vi "Autonomous Independent.vi"   [LabVIEW 2015]
doc: "This VI is called when autonomous begins, and will automatically be terminated when autonomous ends. You can carry out timed or sensor driven robot movement independently without needing to return to the caller."
uses:
  <vilib>/Rock Robotics/WPI/Solenoid/WPI_SolenoidValue.ctl
  <vilib>/Rock Robotics/WPI/Utilities/WPI_GetSetVariantRefNum.vi
  Robot Global Data.vi
  <vilib>/Rock Robotics/WPI/Solenoid/WPI_SolenoidSetEnum.vi
panel:
  # "Be sure to right-click and choose Data Operations>>Make Current Value default if you want to save the array values with the VI"
types:
  T1 = typedef "WPI_JoystickDevRef.ctl" = cluster{"Device":T2}
  T2 = typedef "WPI_JoystickDeviceEnum.ctl" = enum16{"USB 0", "USB 1", "USB 2", "USB 3", "USB 4", "USB 5"}
  T3 = typedef "WPI_SwitchDevRef.ctl" = cluster{"DevStatus":errorcluster, "DIO Channel":T4, "CntIndex":T5, "Normally Closed":bool}
  T4 = typedef "FPGA_DIOChannel.ctl" = enum8{"DIO 0", "DIO 1", "DIO 2", "DIO 3", "DIO 4", "DIO 5", "DIO 6", "DIO 7", "DIO 8", "DIO 9", "DIO MXP 0", "DIO MXP 1", "DIO MXP 2", "DIO MXP 3", "DIO MXP 4", "DIO MXP 5", "DIO MXP 6", "DIO MXP 7", "DIO MXP 8", "DIO MXP 9", "DIO MXP 10", "DIO MXP 11", "DIO MXP 12", "DIO MXP 13", "DIO MXP 14", "DIO MXP 15", "Invalid"}
  T5 = typedef "FPGA_CounterCtrSystemIndex.ctl" = enum8{"Ctr 0", "Ctr 1", "Ctr 2", "Ctr 3", "Ctr 4", "Ctr 5", "Ctr 6", "Ctr 7", "Invalid"}
  T6 = typedef "WPI_SolenoidValue.ctl" = enum16{"Off", "On", "Forward", "Reverse"}
  T7 = enum16{"No pot 1 bin", "3 Tote Spinny", "2 Tote Middle", "1 Bin", "1 Tote", "Drive", "3 Tote"}
  T8 = typedef "WPI_SolenoidDevRef.ctl" = cluster{"DevStatus":errorcluster, "Pneumatics Control Module":u8, "Forward Solenoid Channel":T9, "Reverse Solenoid Channel":T9}
  T9 = typedef "WPI_SolenoidChannel.ctl" = enum8{"Solenoid 0", "Solenoid 1", "Solenoid 2", "Solenoid 3", "Solenoid 4", "Solenoid 5", "Solenoid 6", "Solenoid 7", "Invalid"}
  T10 = typedef "WPI_MotorControlDeviceRef.ctl" = cluster{"DeviceStatus":errorcluster, "Type":T11, "PWM":cluster{"PWM Channel":T12, "DeadBand":T13}, "CAN":cluster{"Device Number":u8, "Control Mode":T14, "Semaphore":T15, "Max Vout":dbl, "TalonSRX Control Mode":T16}, "Invert":bool}
  T11 = typedef "WPI_MotorControlType.ctl" = enum16{"PWM", "CAN", "CANTalonSRX"}
  T12 = typedef "FPGA_DIOPWMChannel.ctl" = enum8{"PWM 0", "PWM 1", "PWM 2", "PWM 3", "PWM 4", "PWM 5", "PWM 6", "PWM 7", "PWM 8", "PWM 9", "PWM MXP 0", "PWM MXP 1", "PWM MXP 2", "PWM MXP 3", "PWM MXP 4", "PWM MXP 5", "PWM MXP 6", "PWM MXP 7", "PWM MXP 8", "PWM MXP 9", "Invalid"}
  T13 = typedef "WPI_PWMDeadband.ctl" = cluster{"Name":string, "maxPositivePwm":i32, "minPositivePwm":i32, "centerPwm":i32, "maxNegativePwm":i32, "minNegativePwm":i32, "angularRange":u16}
  T14 = typedef "WPI_CANJaguar_ControlMode.ctl" = enum8{"Percent VBus", "Current", "Speed", "Position", "Voltage"}
  T15 = typedef "Semaphore RefNum" = refnum<k1>
  T16 = typedef "WPI_CANTalonSRX_APIControlMode.ctl" = enum8{"Percent VBus", "Speed", "Position", "Slave", "Unchanged / Invalid", "Voltage Compensation", "Current", "Motion Profile"}
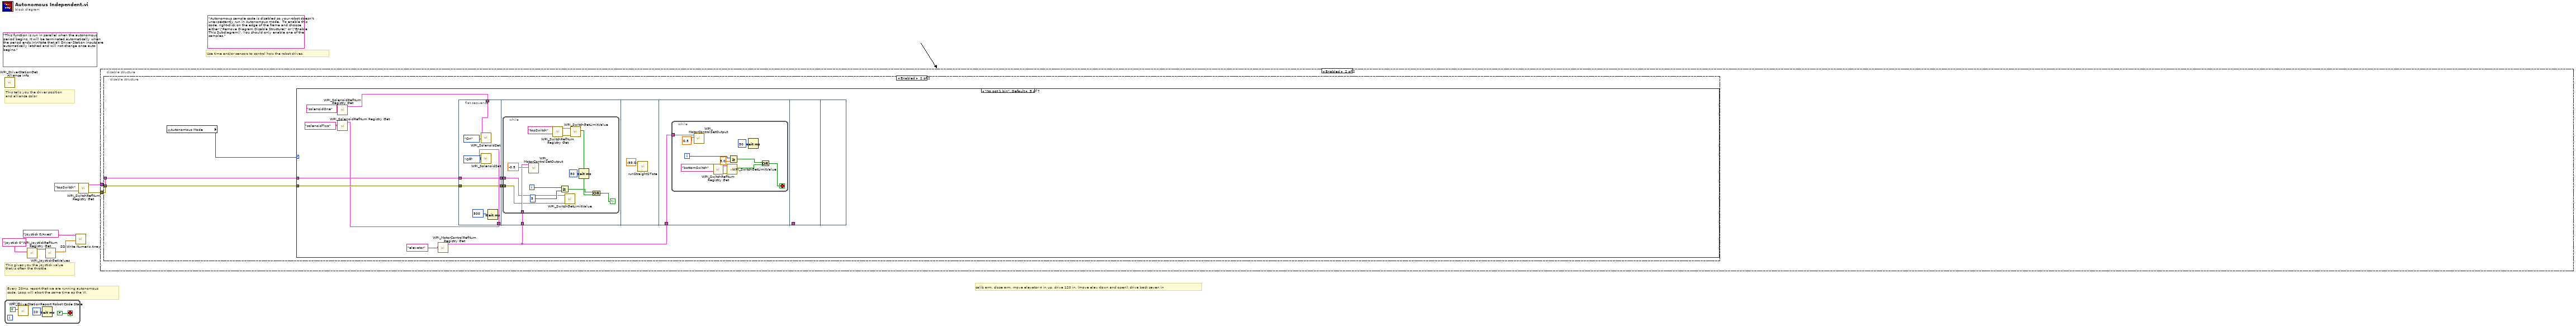
[diagram p0: block diagram]
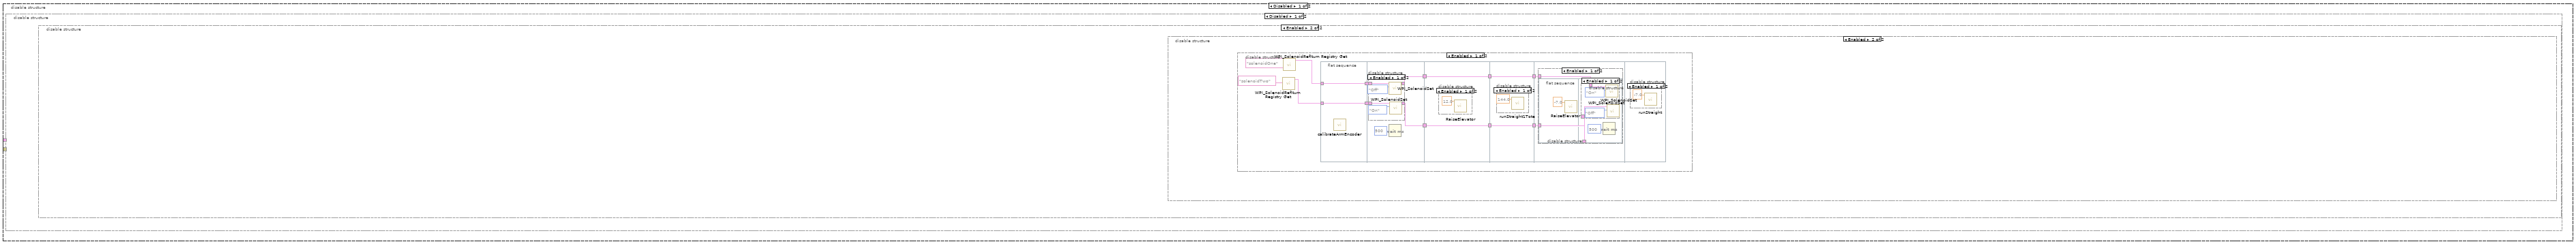
[diagram p2: hidden frame]
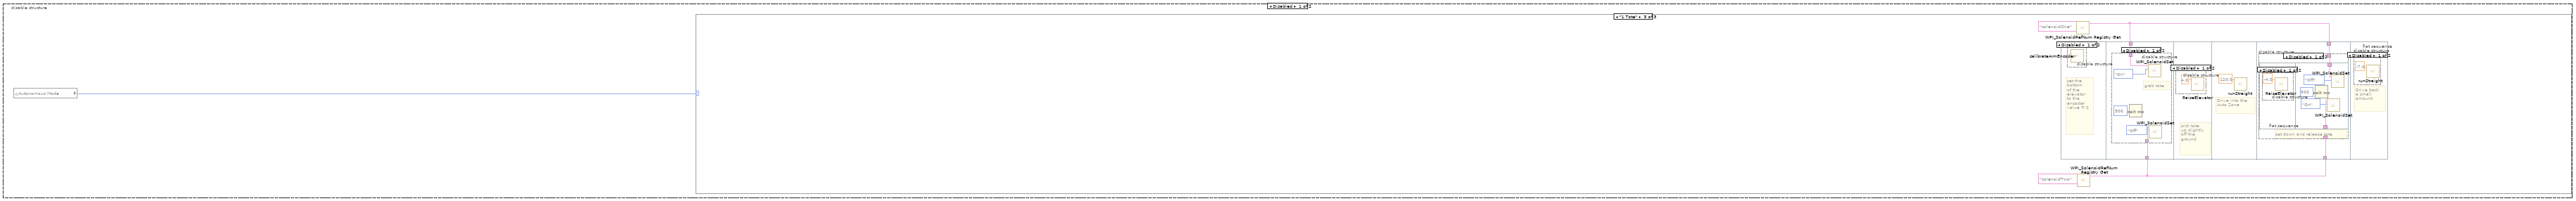
[diagram p3: hidden frame]
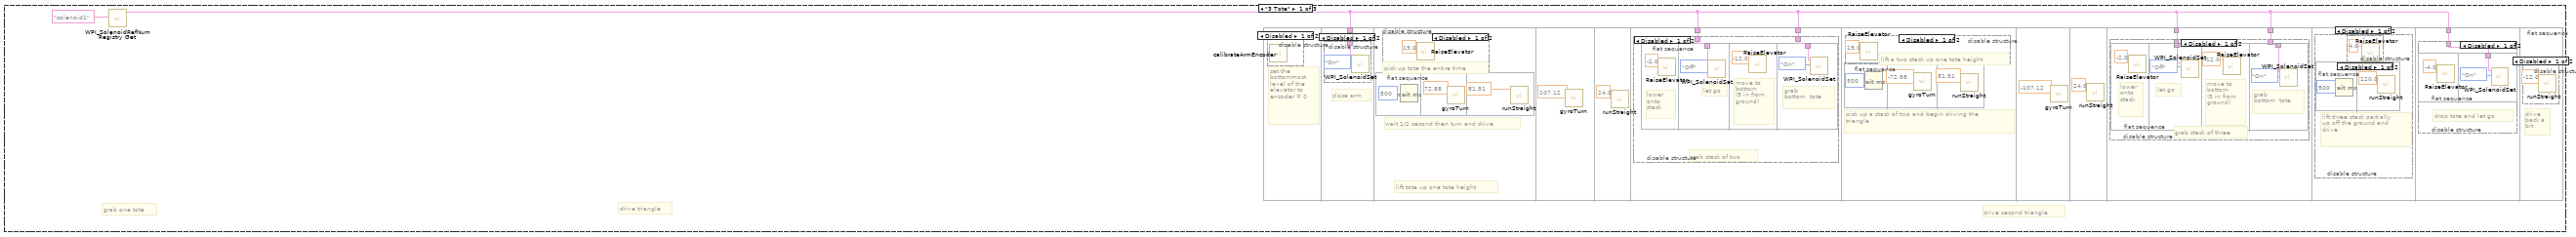
[diagram p4: hidden frame]
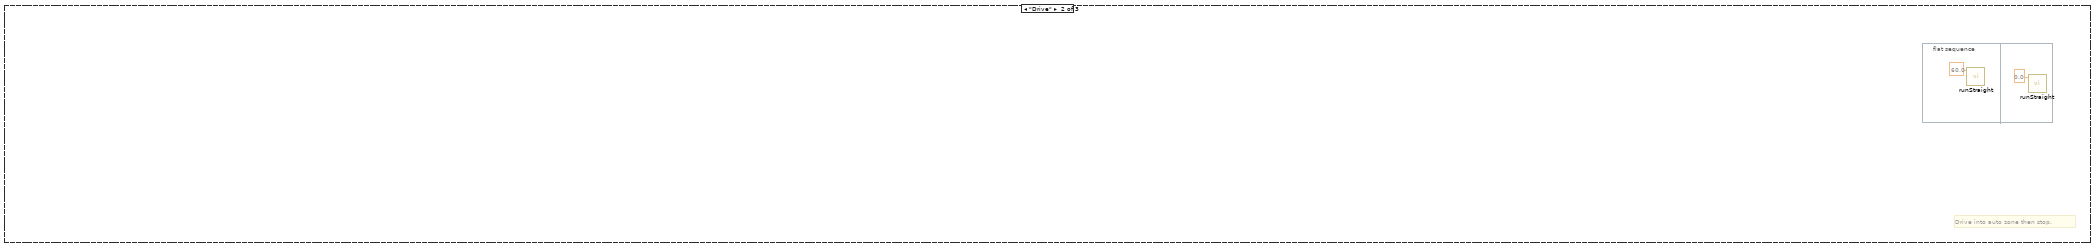
[diagram p15: hidden frame]
diagram:
  (unwired) "Autonomous sample code is disabled so your robot doesn't unexpectantly run in Autonomous mode.  To enable this code, right-click on the edge of the frame and choose either \"Remove Diagram Disable Structure\" or \"Enable This Subdiagram\". You should only enable one of the samples."
  (unwired) "This function is run in parallel when the autonomous period begins. It will be terminated automatically when the period ends.\n\nNote that all Driver Station inputs are automatically latched and will not change once auto begins."
  # "calib arm, close arm, move elevator 4 in up, drive 120 in, (move elev down and open), drive back seven in"
  # "Every 20ms, report that we are running autonomous\ncode. Loop will abort the same time as the VI."
  # "This gives you the joystick value\nthat is often the throttle"
  # "Use time and/or sensors to control how the robot drives."
  # "This tells you the driver position\nand alliance color"
  n1 = while {
    stop <- FALSE stop-if-true
    n2 = call <vilib>:"WPI_DriverStationReport Robot Code State.vi"("Autonomous"=TRUE) -> ()  [unwired: 10 in, 1 out]
    n3 = Wait (ms)(milliseconds to wait=u32 20) -> ()  [unwired: 1 out]
  }
  n4 = call <vilib>:"WPI_DriverStationGet Alliance Info.vi"() -> ()  [unwired: 12 out]
  n5 = call <vilib>:"WPI_JoystickRefNum Registry Get.vi"("refnum name"="Joystick 0") -> ("JoystickDevRef"=w6:T1)  [unwired: 1 in, 9 out]
  n6 = call <vilib>:"WPI_JoystickGetValues.vi"("JoystickDevRef"=w6) -> ("Axes"=w4:dbl[])  [unwired: 6 in, 4 out]
  n7 = call <vilib>:"SD Write Numeric Array.vi"("Numeric Array"=w4, "Name"="Joystick 0/Axes") -> ()  [unwired: 8 in, 2 out]
  n8 = call <vilib>:"WPI_SwitchRefNum Registry Get.vi"("refnum name"="topSwitch") -> ("error out"=w1:errorcluster, "SwitchDevRef"=w2:T3)  [unwired: 9 in]
  n9 = disable-structure shown="Enabled" {
    disable-tunnel: w2 -> [_ w201]
    disable-tunnel: w1 -> [_ w200]
    frame Disabled {
      n10 = disable-structure shown="Disabled" {
        frame Disabled {
          n11 = disable-structure shown="Enabled" {
            frame Disabled {
              n12 = global read "Robot Global Data.vi" "Autonomous Mode"() -> (w11:T7)
              n13 = case shown="\"1 Tote\"" w11 {
                frame "3 Tote" {
                  # "drive triangle"
                  # "drive second triangle"
                  # "grab one tote"
                  n14 = call <vilib>:"WPI_SolenoidRefNum Registry Get.vi"("refnum name"="solenoid1") -> ("SolenoidDevRef"=w13:T8)  [unwired: 9 in, 1 out]
                  n15 = flat-sequence {
                    tunnel: w13 -> [w14]
                    tunnel: w13 -> [w24]
                    tunnel: w13 -> [w23]
                    tunnel: w13 -> [w40]
                    tunnel: w13 -> [w39]
                    tunnel: w13 -> [w52]
                    frame #0 {
                      # "set the \nbottommost\nlevel of the \nelevator to \nencoder = 0"
                      n16 = disable-structure shown="Disabled" {
                        frame Disabled {
                          n17 = call "calibrateArmEncoder.vi"() -> ()  [unwired: 12 in]
                        }
                        frame Enabled {
                        }
                      }
                    }
                    frame #1 {
                      # "close arm"
                      n18 = disable-structure shown="Disabled" {
                        disable-tunnel: w14 -> [w15 _]
                        frame Disabled {
                          n19 = call-poly <vilib>:"WPI_SolenoidSet.vi"("Value"=WPI_SolenoidValue."On", "SolenoidDevRef"=w15) -> ()  [unwired: 8 in, 2 out]
                        }
                        frame Enabled {
                        }
                      }
                    }
                    frame #2 {
                      # "lift tote up one tote height"
                      # "wait 1/2 second then turn and drive"
                      n20 = flat-sequence {
                        frame #0 {
                          n21 = Wait (ms)(milliseconds to wait=u32 500) -> ()  [unwired: 1 out]
                        }
                        frame #1 {
                          n22 = call "gyroTurn.vi"("Angle"=72.88) -> ()  [unwired: 11 in]
                        }
                        frame #2 {
                          n23 = call "runStraight.vi"("Distance In"=81.51) -> ()  [unwired: 11 in]
                        }
                      }
                      n24 = disable-structure shown="Disabled" {
                        frame Disabled {
                          # "pick up tote the entire time"
                          n25 = call "RaiseElevator.vi"("Distance"=19.0) -> ()  [unwired: 11 in]
                        }
                        frame Enabled {
                        }
                      }
                    }
                    frame #3 {
                      n26 = call "gyroTurn.vi"("Angle"=107.12) -> ()  [unwired: 11 in]
                    }
                    frame #4 {
                      n27 = call "runStraight.vi"("Distance In"=24.0) -> ()  [unwired: 11 in]
                    }
                    frame #5 {
                      n28 = disable-structure shown="Disabled" {
                        disable-tunnel: w24 -> [w26 _]
                        disable-tunnel: w23 -> [w25 _]
                        frame Disabled {
                          # "grab stack of two"
                          n29 = flat-sequence {
                            tunnel: w26 -> [w28]
                            tunnel: w25 -> [w31]
                            frame #0 {
                              # "lower onto\nstack"
                              n30 = call "RaiseElevator.vi"("Distance"=-2.0) -> ()  [unwired: 11 in]
                            }
                            frame #1 {
                              # "let go"
                              n31 = call-poly <vilib>:"WPI_SolenoidSet.vi"("Value"=WPI_SolenoidValue."Off", "SolenoidDevRef"=w28) -> ()  [unwired: 8 in, 2 out]
                            }
                            frame #2 {
                              # "move to\nbottom \n(5 in from\nground)"
                              n32 = call "RaiseElevator.vi"("Distance"=-12.0) -> ()  [unwired: 11 in]
                            }
                            frame #3 {
                              # "grab \nbottom  tote"
                              n33 = call-poly <vilib>:"WPI_SolenoidSet.vi"("Value"=WPI_SolenoidValue."On", "SolenoidDevRef"=w31) -> ()  [unwired: 8 in, 2 out]
                            }
                          }
                        }
                        frame Enabled {
                        }
                      }
                    }
                    frame #6 {
                      # "pick up a stack of two and begin driving the \ntriangle"
                      n34 = flat-sequence {
                        frame #0 {
                          n35 = Wait (ms)(milliseconds to wait=u32 500) -> ()  [unwired: 1 out]
                        }
                        frame #1 {
                          n36 = call "gyroTurn.vi"("Angle"=-72.88) -> ()  [unwired: 11 in]
                        }
                        frame #2 {
                          n37 = call "runStraight.vi"("Distance In"=81.51) -> ()  [unwired: 11 in]
                        }
                      }
                      n38 = disable-structure shown="Disabled" {
                        frame Disabled {
                          # "lift a two stack up one tote height"
                          n39 = call "RaiseElevator.vi"("Distance"=19.0) -> ()  [unwired: 11 in]
                        }
                        frame Enabled {
                        }
                      }
                    }
                    frame #7 {
                      n40 = call "gyroTurn.vi"("Angle"=-107.12) -> ()  [unwired: 11 in]
                    }
                    frame #8 {
                      n41 = call "runStraight.vi"("Distance In"=24.0) -> ()  [unwired: 11 in]
                    }
                    frame #9 {
                      n42 = disable-structure shown="Disabled" {
                        disable-tunnel: w40 -> [w42 _]
                        disable-tunnel: w39 -> [w41 _]
                        frame Disabled {
                          # "grab stack of three"
                          n43 = flat-sequence {
                            tunnel: w42 -> [w44]
                            tunnel: w41 -> [w47]
                            frame #0 {
                              # "lower\nonto\nstack"
                              n44 = call "RaiseElevator.vi"("Distance"=-2.0) -> ()  [unwired: 11 in]
                            }
                            frame #1 {
                              # "let go"
                              n45 = call-poly <vilib>:"WPI_SolenoidSet.vi"("Value"=WPI_SolenoidValue."Off", "SolenoidDevRef"=w44) -> ()  [unwired: 8 in, 2 out]
                            }
                            frame #2 {
                              # "move to\nbottom \n(5 in from\nground)"
                              n46 = call "RaiseElevator.vi"("Distance"=-12.0) -> ()  [unwired: 11 in]
                            }
                            frame #3 {
                              # "grab \nbottom  tote"
                              n47 = call-poly <vilib>:"WPI_SolenoidSet.vi"("Value"=WPI_SolenoidValue."On", "SolenoidDevRef"=w47) -> ()  [unwired: 8 in, 2 out]
                            }
                          }
                        }
                        frame Enabled {
                        }
                      }
                    }
                    frame #10 {
                      n48 = disable-structure shown="Disabled" {
                        frame Disabled {
                          # "lift three stack partially \nup off the ground and \ndrive"
                          n49 = flat-sequence {
                            frame #0 {
                              n50 = Wait (ms)(milliseconds to wait=u32 500) -> ()  [unwired: 1 out]
                            }
                            frame #1 {
                              n51 = call "runStraight.vi"("Distance In"=120.0) -> ()  [unwired: 11 in]
                            }
                          }
                          n52 = disable-structure shown="Disabled" {
                            frame Disabled {
                              n53 = call "RaiseElevator.vi"("Distance"=4.0) -> ()  [unwired: 11 in]
                            }
                            frame Enabled {
                            }
                          }
                        }
                        frame Enabled {
                        }
                      }
                    }
                    frame #11 {
                      n54 = disable-structure shown="Disabled" {
                        disable-tunnel: w52 -> [w53 _]
                        frame Disabled {
                          # "drop tote and let go"
                          n55 = flat-sequence {
                            tunnel: w53 -> [w55]
                            frame #0 {
                              n56 = call "RaiseElevator.vi"("Distance"=-4.0) -> ()  [unwired: 11 in]
                            }
                            frame #1 {
                              n57 = call-poly <vilib>:"WPI_SolenoidSet.vi"("Value"=WPI_SolenoidValue."On", "SolenoidDevRef"=w55) -> ()  [unwired: 8 in, 2 out]
                            }
                          }
                        }
                        frame Enabled {
                        }
                      }
                    }
                    frame #12 {
                      # "drive \nback a \nbit"
                      n58 = disable-structure shown="Disabled" {
                        frame Disabled {
                          n59 = call "runStraight.vi"("Distance In"=-12.0) -> ()  [unwired: 11 in]
                        }
                        frame Enabled {
                        }
                      }
                    }
                  }
                }
                frame "Drive" {
                  # "Drive into auto zone then stop."
                  n60 = flat-sequence {
                    frame #0 {
                      n61 = call "runStraight.vi"("Distance In"=60.0) -> ()  [unwired: 11 in]
                    }
                    frame #1 {
                      n62 = call "runStraight.vi"("Distance In"=0.0) -> ()  [unwired: 11 in]
                    }
                  }
                }
                frame "1 Tote" {
                  n63 = flat-sequence {
                    tunnel: w62 -> [w65]
                    tunnel: w60 -> [w64]
                    tunnel: w62 -> [w74]
                    tunnel: w60 -> [w73]
                    frame #0 {
                      # "set the \nbottom\nof the\nelevator\nto the\nencoder\nvalue = 0"
                      n64 = disable-structure shown="Disabled" {
                        frame Disabled {
                          n65 = call "calibrateArmEncoder.vi"() -> ()  [unwired: 12 in]
                        }
                        frame Enabled {
                        }
                      }
                    }
                    frame #1 {
                      n66 = disable-structure shown="Disabled" {
                        disable-tunnel: w65 -> [w70 _]
                        disable-tunnel: w64 -> [w67 _]
                        frame Disabled {
                          # "grab tote"
                          n67 = Wait (ms)(milliseconds to wait=u32 500) -> ()  [unwired: 1 out]
                          n68 = call-poly <vilib>:"WPI_SolenoidSet.vi"("Value"=WPI_SolenoidValue."On", "SolenoidDevRef"=w70) -> ()  [unwired: 8 in, 2 out]
                          n69 = call-poly <vilib>:"WPI_SolenoidSet.vi"("Value"=WPI_SolenoidValue."Off", "SolenoidDevRef"=w67) -> ()  [unwired: 8 in, 2 out]
                        }
                        frame Enabled {
                        }
                      }
                    }
                    frame #2 {
                      # "pick tote\nup slightly\noff the \nground"
                      n70 = disable-structure shown="Disabled" {
                        frame Disabled {
                          n71 = call "RaiseElevator.vi"("Distance"=4.0) -> ()  [unwired: 11 in]
                        }
                        frame Enabled {
                        }
                      }
                    }
                    frame #3 {
                      # "Drive into the\nAuto Zone"
                      n72 = call "runStraight.vi"("Distance In"=120.0) -> ()  [unwired: 11 in]
                    }
                    frame #4 {
                      n73 = disable-structure shown="Disabled" {
                        disable-tunnel: w74 -> [w76 _]
                        disable-tunnel: w73 -> [w75 _]
                        frame Disabled {
                          # "set down and release tote"
                          n74 = flat-sequence {
                            tunnel: w76 -> [w81]
                            tunnel: w75 -> [w79]
                            frame #0 {
                              n75 = disable-structure shown="Disabled" {
                                frame Disabled {
                                n76 = call "RaiseElevator.vi"("Distance"=-4.0) -> ()  [unwired: 11 in]
                                }
                                frame Enabled {
                                }
                              }
                            }
                            frame #1 {
                              n77 = Wait (ms)(milliseconds to wait=u32 500) -> ()  [unwired: 1 out]
                              n78 = call-poly <vilib>:"WPI_SolenoidSet.vi"("Value"=WPI_SolenoidValue."On", "SolenoidDevRef"=w79) -> ()  [unwired: 8 in, 2 out]
                              n79 = call-poly <vilib>:"WPI_SolenoidSet.vi"("Value"=WPI_SolenoidValue."Off", "SolenoidDevRef"=w81) -> ()  [unwired: 8 in, 2 out]
                            }
                          }
                        }
                        frame Enabled {
                        }
                      }
                    }
                    frame #5 {
                      # "Drive back\na small \namount"
                      n80 = disable-structure shown="Disabled" {
                        frame Disabled {
                          n81 = call "runStraight.vi"("Distance In"=-7.0) -> ()  [unwired: 11 in]
                        }
                        frame Enabled {
                        }
                      }
                    }
                  }
                  n82 = call <vilib>:"WPI_SolenoidRefNum Registry Get.vi"("refnum name"="solenoidOne") -> ("SolenoidDevRef"=w62:T8)  [unwired: 9 in, 1 out]
                  n83 = call <vilib>:"WPI_SolenoidRefNum Registry Get.vi"("refnum name"="solenoidTwo") -> ("SolenoidDevRef"=w60:T8)  [unwired: 9 in, 1 out]
                }
              }
            }
            frame Enabled {
              n84 = disable-structure shown="Enabled" {
                frame Disabled {
                  # "drive triangle"
                  # "drive second triangle"
                  # "grab one tote"
                  n85 = call <vilib>:"WPI_SolenoidRefNum Registry Get.vi"("refnum name"="solenoid1") -> ("SolenoidDevRef"=w85:T8)  [unwired: 9 in, 1 out]
                  n86 = flat-sequence {
                    tunnel: w85 -> [w86]
                    tunnel: w85 -> [w96]
                    tunnel: w85 -> [w95]
                    tunnel: w85 -> [w112]
                    tunnel: w85 -> [w111]
                    tunnel: w85 -> [w124]
                    frame #0 {
                      # "set the \nbottommost\nlevel of the \nelevator to \nencoder = 0"
                      n87 = disable-structure shown="Disabled" {
                        frame Disabled {
                          n88 = call "calibrateArmEncoder.vi"() -> ()  [unwired: 12 in]
                        }
                        frame Enabled {
                        }
                      }
                    }
                    frame #1 {
                      # "close arm"
                      n89 = disable-structure shown="Disabled" {
                        disable-tunnel: w86 -> [w87 _]
                        frame Disabled {
                          n90 = call-poly <vilib>:"WPI_SolenoidSet.vi"("Value"=WPI_SolenoidValue."On", "SolenoidDevRef"=w87) -> ()  [unwired: 8 in, 2 out]
                        }
                        frame Enabled {
                        }
                      }
                    }
                    frame #2 {
                      # "lift tote up one tote height"
                      # "wait 1/2 second then turn and drive"
                      n91 = flat-sequence {
                        frame #0 {
                          n92 = Wait (ms)(milliseconds to wait=u32 500) -> ()  [unwired: 1 out]
                        }
                        frame #1 {
                          n93 = call "gyroTurn.vi"("Angle"=-72.88) -> ()  [unwired: 11 in]
                        }
                        frame #2 {
                          n94 = call "runStraight.vi"("Distance In"=81.51) -> ()  [unwired: 11 in]
                        }
                      }
                      n95 = disable-structure shown="Disabled" {
                        frame Disabled {
                          # "pick up tote the entire time"
                          n96 = call "RaiseElevator.vi"("Distance"=19.0) -> ()  [unwired: 11 in]
                        }
                        frame Enabled {
                        }
                      }
                    }
                    frame #3 {
                      n97 = call "gyroTurn.vi"("Angle"=-107.12) -> ()  [unwired: 11 in]
                    }
                    frame #4 {
                      n98 = call "runStraight.vi"("Distance In"=24.0) -> ()  [unwired: 11 in]
                    }
                    frame #5 {
                      n99 = disable-structure shown="Disabled" {
                        disable-tunnel: w96 -> [w98 _]
                        disable-tunnel: w95 -> [w97 _]
                        frame Disabled {
                          # "grab stack of two"
                          n100 = flat-sequence {
                            tunnel: w98 -> [w100]
                            tunnel: w97 -> [w103]
                            frame #0 {
                              # "lower onto\nstack"
                              n101 = call "RaiseElevator.vi"("Distance"=-2.0) -> ()  [unwired: 11 in]
                            }
                            frame #1 {
                              # "let go"
                              n102 = call-poly <vilib>:"WPI_SolenoidSet.vi"("Value"=WPI_SolenoidValue."Off", "SolenoidDevRef"=w100) -> ()  [unwired: 8 in, 2 out]
                            }
                            frame #2 {
                              # "move to\nbottom \n(5 in from\nground)"
                              n103 = call "RaiseElevator.vi"("Distance"=-12.0) -> ()  [unwired: 11 in]
                            }
                            frame #3 {
                              # "grab \nbottom  tote"
                              n104 = call-poly <vilib>:"WPI_SolenoidSet.vi"("Value"=WPI_SolenoidValue."On", "SolenoidDevRef"=w103) -> ()  [unwired: 8 in, 2 out]
                            }
                          }
                        }
                        frame Enabled {
                        }
                      }
                    }
                    frame #6 {
                      # "pick up a stack of two and begin driving the \ntriangle"
                      n105 = flat-sequence {
                        frame #0 {
                          n106 = Wait (ms)(milliseconds to wait=u32 500) -> ()  [unwired: 1 out]
                        }
                        frame #1 {
                          n107 = call "gyroTurn.vi"("Angle"=72.88) -> ()  [unwired: 11 in]
                        }
                        frame #2 {
                          n108 = call "runStraight.vi"("Distance In"=81.51) -> ()  [unwired: 11 in]
                        }
                      }
                      n109 = disable-structure shown="Disabled" {
                        frame Disabled {
                          # "lift a two stack up one tote height"
                          n110 = call "RaiseElevator.vi"("Distance"=19.0) -> ()  [unwired: 11 in]
                        }
                        frame Enabled {
                        }
                      }
                    }
                    frame #7 {
                      n111 = call "gyroTurn.vi"("Angle"=107.12) -> ()  [unwired: 11 in]
                    }
                    frame #8 {
                      n112 = call "runStraight.vi"("Distance In"=24.0) -> ()  [unwired: 11 in]
                    }
                    frame #9 {
                      n113 = disable-structure shown="Disabled" {
                        disable-tunnel: w112 -> [w114 _]
                        disable-tunnel: w111 -> [w113 _]
                        frame Disabled {
                          # "grab stack of three"
                          n114 = flat-sequence {
                            tunnel: w114 -> [w116]
                            tunnel: w113 -> [w119]
                            frame #0 {
                              # "lower\nonto\nstack"
                              n115 = call "RaiseElevator.vi"("Distance"=-2.0) -> ()  [unwired: 11 in]
                            }
                            frame #1 {
                              # "let go"
                              n116 = call-poly <vilib>:"WPI_SolenoidSet.vi"("Value"=WPI_SolenoidValue."Off", "SolenoidDevRef"=w116) -> ()  [unwired: 8 in, 2 out]
                            }
                            frame #2 {
                              # "move to\nbottom \n(5 in from\nground)"
                              n117 = call "RaiseElevator.vi"("Distance"=-12.0) -> ()  [unwired: 11 in]
                            }
                            frame #3 {
                              # "grab \nbottom  tote"
                              n118 = call-poly <vilib>:"WPI_SolenoidSet.vi"("Value"=WPI_SolenoidValue."On", "SolenoidDevRef"=w119) -> ()  [unwired: 8 in, 2 out]
                            }
                          }
                        }
                        frame Enabled {
                        }
                      }
                    }
                    frame #10 {
                      n119 = disable-structure shown="Disabled" {
                        frame Disabled {
                          # "lift three stack partially \nup off the ground and \ndrive"
                          n120 = flat-sequence {
                            frame #0 {
                              n121 = Wait (ms)(milliseconds to wait=u32 500) -> ()  [unwired: 1 out]
                            }
                            frame #1 {
                              n122 = call "runStraight.vi"("Distance In"=120.0) -> ()  [unwired: 11 in]
                            }
                          }
                          n123 = disable-structure shown="Disabled" {
                            frame Disabled {
                              n124 = call "RaiseElevator.vi"("Distance"=4.0) -> ()  [unwired: 11 in]
                            }
                            frame Enabled {
                            }
                          }
                        }
                        frame Enabled {
                        }
                      }
                    }
                    frame #11 {
                      n125 = disable-structure shown="Disabled" {
                        disable-tunnel: w124 -> [w125 _]
                        frame Disabled {
                          # "drop tote and let go"
                          n126 = flat-sequence {
                            tunnel: w125 -> [w127]
                            frame #0 {
                              n127 = call "RaiseElevator.vi"("Distance"=-4.0) -> ()  [unwired: 11 in]
                            }
                            frame #1 {
                              n128 = call-poly <vilib>:"WPI_SolenoidSet.vi"("Value"=WPI_SolenoidValue."On", "SolenoidDevRef"=w127) -> ()  [unwired: 8 in, 2 out]
                            }
                          }
                        }
                        frame Enabled {
                        }
                      }
                    }
                    frame #12 {
                      # "drive \nback a \nbit"
                      n129 = disable-structure shown="Disabled" {
                        frame Disabled {
                          n130 = call "runStraight.vi"("Distance In"=-12.0) -> ()  [unwired: 11 in]
                        }
                        frame Enabled {
                        }
                      }
                    }
                  }
                }
                frame Enabled {
                  n131 = disable-structure shown="Enabled" {
                    frame Enabled {
                      n132 = call <vilib>:"WPI_SolenoidRefNum Registry Get.vi"("refnum name"="solenoidTwo") -> ("SolenoidDevRef"=w132:T8)  [unwired: 9 in, 1 out]
                      n133 = call <vilib>:"WPI_SolenoidRefNum Registry Get.vi"("refnum name"="solenoidOne") -> ("SolenoidDevRef"=w133:T8)  [unwired: 9 in, 1 out]
                      n134 = flat-sequence {
                        tunnel: w132 -> [w142]
                        tunnel: w133 -> [w143]
                        tunnel: [w143] -> w141
                        tunnel: [w142] -> w140
                        tunnel: [w146] -> w139
                        tunnel: [w145] -> w138
                        tunnel: w141 -> [w148]
                        tunnel: w140 -> [w147]
                        tunnel: [w156] -> w137
                        tunnel: w139 -> [w156]
                        tunnel: [w155] -> w136
                        tunnel: w138 -> [w155]
                        tunnel: [w159] -> w135
                        tunnel: w137 -> [w159]
                        tunnel: [w158] -> w134
                        tunnel: w136 -> [w158]
                        tunnel: w135 -> [w162]
                        tunnel: w134 -> [w161]
                        frame #0 {
                          n135 = call "calibrateArmEncoder.vi"() -> ()  [unwired: 12 in]
                        }
                        frame #1 {
                          n136 = disable-structure shown="Enabled" {
                            disable-tunnel: w148 -> [w154 _]
                            disable-tunnel: w147 -> [w153 _]
                            disable-tunnel: [w150 _] -> w146
                            disable-tunnel: [w149 _] -> w145
                            frame Enabled {
                              n137 = call-poly <vilib>:"WPI_SolenoidSet.vi"("Value"=WPI_SolenoidValue."Off", "SolenoidDevRef"=w154) -> ("SolenoidDevRef"=w150:T8)  [unwired: 8 in, 1 out]
                              n138 = call-poly <vilib>:"WPI_SolenoidSet.vi"("Value"=WPI_SolenoidValue."On", "SolenoidDevRef"=w153) -> ("SolenoidDevRef"=w149:T8)  [unwired: 8 in, 1 out]
                            }
                            frame Disabled {
                            }
                          }
                          n139 = Wait (ms)(milliseconds to wait=u32 500) -> ()  [unwired: 1 out]
                        }
                        frame #2 {
                          n140 = disable-structure shown="Enabled" {
                            frame Enabled {
                              n141 = call "RaiseElevator.vi"("Distance"=12.0) -> ()  [unwired: 11 in]
                            }
                            frame Disabled {
                            }
                          }
                        }
                        frame #3 {
                          n142 = disable-structure shown="Enabled" {
                            frame Enabled {
                              n143 = call "runStraight1Tote.vi"("Distance In"=144.0) -> ()  [unwired: 11 in]
                            }
                            frame Disabled {
                            }
                          }
                        }
                        frame #4 {
                          n144 = disable-structure shown="Enabled" {
                            disable-tunnel: w162 -> [w164 _]
                            disable-tunnel: w161 -> [w163 _]
                            frame Enabled {
                              n145 = flat-sequence {
                                tunnel: w164 -> [w168]
                                tunnel: w163 -> [w167]
                                frame #0 {
                                n146 = call "RaiseElevator.vi"("Distance"=-7.0) -> ()  [unwired: 11 in]
                                }
                                frame #1 {
                                n147 = disable-structure shown="Enabled" {
                                disable-tunnel: w168 -> [w170 _]
                                disable-tunnel: w167 -> [w169 _]
                                frame Enabled {
                                n148 = call-poly <vilib>:"WPI_SolenoidSet.vi"("Value"=WPI_SolenoidValue."On", "SolenoidDevRef"=w170) -> ()  [unwired: 8 in, 2 out]
                                n149 = call-poly <vilib>:"WPI_SolenoidSet.vi"("Value"=WPI_SolenoidValue."Off", "SolenoidDevRef"=w169) -> ()  [unwired: 8 in, 2 out]
                                }
                                frame Disabled {
                                }
                                }
                                n150 = Wait (ms)(milliseconds to wait=u32 500) -> ()  [unwired: 1 out]
                                }
                              }
                            }
                            frame Disabled {
                            }
                          }
                        }
                        frame #5 {
                          n151 = disable-structure shown="Enabled" {
                            frame Enabled {
                              n152 = call "runStraight.vi"("Distance In"=-7.0) -> ()  [unwired: 11 in]
                            }
                            frame Disabled {
                            }
                          }
                        }
                      }
                    }
                    frame Disabled {
                      n153 = flat-sequence {
                        frame #0 {
                          n154 = call "gyroTurn.vi"("Angle"=90.0) -> ()  [unwired: 11 in]
                        }
                      }
                    }
                  }
                }
              }
            }
          }
        }
        frame Enabled {
          n155 = call <vilib>:"WPI_SolenoidRefNum Registry Get.vi"("refnum name"="solenoidTwo") -> ("SolenoidDevRef"=w176:T8)  [unwired: 9 in, 1 out]
          n156 = call <vilib>:"WPI_SolenoidRefNum Registry Get.vi"("refnum name"="solenoidOne") -> ("SolenoidDevRef"=w175:T8)  [unwired: 9 in, 1 out]
          n157 = flat-sequence {
            tunnel: w176 -> [w185]
            tunnel: w175 -> [w184]
            tunnel: w175 -> [w192]
            tunnel: w176 -> [w191]
            frame #0 {
              n158 = call "calibrateArmEncoder.vi"() -> ()  [unwired: 12 in]
            }
            frame #1 {
              # "raise elevator"
              n159 = call "RaiseElevator.vi"("Distance"=14.0) -> ()  [unwired: 11 in]
            }
            frame #2 {
              n160 = call "runStraight1Tote.vi"("Distance In"=18.0) -> ()  [unwired: 11 in]
            }
            frame #3 {
              n161 = call "runStraight1Tote.vi"("Distance In"=-6.0) -> ()  [unwired: 11 in]
            }
            frame #4 {
              # "lower elevator"
              n162 = call "RaiseElevator.vi"("Distance"=-14.0) -> ()  [unwired: 11 in]
            }
            frame #5 {
              # "drive forward 6"
              n163 = call "runStraight1Tote.vi"("Distance In"=6.0) -> ()  [unwired: 11 in]
            }
            frame #6 {
              n164 = Wait (ms)(milliseconds to wait=u32 500) -> ()  [unwired: 1 out]
              n165 = call-poly <vilib>:"WPI_SolenoidSet.vi"("Value"=WPI_SolenoidValue."Off", "SolenoidDevRef"=w184) -> ()  [unwired: 8 in, 2 out]
              n166 = call-poly <vilib>:"WPI_SolenoidSet.vi"("Value"=WPI_SolenoidValue."On", "SolenoidDevRef"=w185) -> ()  [unwired: 8 in, 2 out]
            }
            frame #7 {
              n167 = call "RaiseElevator.vi"("Distance"=12.0) -> ()  [unwired: 11 in]
            }
            frame #8 {
              n168 = call "runStraight1Tote.vi"("Distance In"=-162.0) -> ()  [unwired: 11 in]
            }
            frame #9 {
              n169 = flat-sequence {
                tunnel: w192 -> [w198]
                tunnel: w191 -> [w197]
                frame #0 {
                  n170 = call "RaiseElevator.vi"("Distance"=-7.0) -> ()  [unwired: 11 in]
                }
                frame #1 {
                  n171 = Wait (ms)(milliseconds to wait=u32 500) -> ()  [unwired: 1 out]
                  n172 = call-poly <vilib>:"WPI_SolenoidSet.vi"("Value"=WPI_SolenoidValue."On", "SolenoidDevRef"=w198) -> ()  [unwired: 8 in, 2 out]
                  n173 = call-poly <vilib>:"WPI_SolenoidSet.vi"("Value"=WPI_SolenoidValue."Off", "SolenoidDevRef"=w197) -> ()  [unwired: 8 in, 2 out]
                }
              }
            }
            frame #10 {
              n174 = call "runStraight.vi"("Distance In"=-7.0) -> ()  [unwired: 11 in]
            }
          }
        }
      }
    }
    frame Enabled {
      n175 = disable-structure shown="Enabled" {
        disable-tunnel: w201 -> [_ w246]
        disable-tunnel: w200 -> [_ w245]
        frame Disabled {
          n176 = disable-structure shown="Enabled" {
            frame Disabled {
              n177 = flat-sequence {
                frame #0 {
                  n178 = call "calibrateArmEncoder.vi"() -> ()  [unwired: 12 in]
                }
                frame #1 {
                  n179 = call "RaiseElevator.vi"("Distance"=6.0) -> ()  [unwired: 11 in]
                }
                frame #2 {
                  n180 = Wait (ms)(milliseconds to wait=u32 2000) -> ()  [unwired: 1 out]
                }
                frame #3 {
                  n181 = call "RaiseElevator.vi"("Distance"=-3.0) -> ()  [unwired: 11 in]
                }
                frame #4 {
                  n182 = Wait (ms)(milliseconds to wait=u32 2000) -> ()  [unwired: 1 out]
                }
                frame #5 {
                  n183 = call "RaiseElevator.vi"("Distance"=9.0) -> ()  [unwired: 11 in]
                }
                frame #6 {
                  n184 = Wait (ms)(milliseconds to wait=u32 2000) -> ()  [unwired: 1 out]
                }
                frame #7 {
                  n185 = call "RaiseElevator.vi"("Distance"=-2.0) -> ()  [unwired: 11 in]
                }
              }
            }
            frame Enabled {
              n186 = call <vilib>:"WPI_SolenoidRefNum Registry Get.vi"("refnum name"="solenoidOne") -> ("SolenoidDevRef"=w211:T8)  [unwired: 9 in, 1 out]
              n187 = call <vilib>:"WPI_SolenoidRefNum Registry Get.vi"("refnum name"="solenoidTwo") -> ("SolenoidDevRef"=w212:T8)  [unwired: 9 in, 1 out]
              n188 = call <vilib>:"WPI_MotorControlRefNum Registry Get.vi"("refnum name"="elevator") -> ("MotorControlDevRef"=w209:T10)  [unwired: 9 in, 1 out]
              n189 = flat-sequence {
                tunnel: w211 -> [_]
                tunnel: w212 -> [_]
                tunnel: w211 -> [w218]
                tunnel: w212 -> [w216]
                tunnel: w209 -> [w220]
                tunnel: w209 -> [w233]
                tunnel: w212 -> [_]
                tunnel: w211 -> [_]
                frame #0 {
                }
                frame #1 {
                }
                frame #2 {
                }
                frame #3 {
                  n190 = call-poly <vilib>:"WPI_SolenoidSet.vi"("Value"=WPI_SolenoidValue."On", "SolenoidDevRef"=w218) -> ()  [unwired: 8 in, 2 out]
                  n191 = Wait (ms)(milliseconds to wait=u32 500) -> ()  [unwired: 1 out]
                  n192 = call-poly <vilib>:"WPI_SolenoidSet.vi"("Value"=WPI_SolenoidValue."Off", "SolenoidDevRef"=w216) -> ()  [unwired: 8 in, 2 out]
                }
                frame #4 {
                  n193 = while {
                    tunnel: w220 -> [w231]
                    i -> [w222]
                    stop <- w224 stop-if-true
                    n194 = call <vilib>:"WPI_MotorControlSetOutput.vi"("Output"=-0.5, "MotorControlDevRef"=w231) -> ()  [unwired: 7 in, 3 out]
                    n195 = call <vilib>:"WPI_SwitchRefNum Registry Get.vi"("refnum name"="topSwitch") -> ("error out"=w229:errorcluster, "SwitchDevRef"=w228:T3)  [unwired: 9 in]
                    n196 = call <vilib>:"WPI_SwitchGetLimitValue.vi"("error in (no error)"=w229, "SwitchDevRef"=w228) -> ("Switch Pressed"=w226:bool)  [unwired: 7 in, 2 out]
                    n197 = Greater Or Equal?(x=w222, y=5.0) -> (x >= y?=w225:bool)
                    n198 = Wait (ms)(milliseconds to wait=u32 50) -> ()  [unwired: 1 out]
                    n199 = Or(x=w225, y=w226) -> (x .or. y?=w224:bool)
                  }
                }
                frame #5 {
                  n200 = call "runStraight1Tote.vi"("Distance In"=-70.0) -> ()  [unwired: 11 in]
                }
                frame #6 {
                  n201 = while {
                    tunnel: w233 -> [w244]
                    i -> [w235]
                    stop <- w237 stop-if-true
                    n202 = call <vilib>:"WPI_MotorControlSetOutput.vi"("Output"=0.5, "MotorControlDevRef"=w244) -> ()  [unwired: 7 in, 3 out]
                    n203 = call <vilib>:"WPI_SwitchRefNum Registry Get.vi"("refnum name"="bottomSwitch") -> ("error out"=w242:errorcluster, "SwitchDevRef"=w241:T3)  [unwired: 9 in]
                    n204 = call <vilib>:"WPI_SwitchGetLimitValue.vi"("error in (no error)"=w242, "SwitchDevRef"=w241) -> ("Switch Pressed"=w239:bool)  [unwired: 7 in, 2 out]
                    n205 = Greater Or Equal?(x=w235, y=5.0) -> (x >= y?=w238:bool)
                    n206 = Wait (ms)(milliseconds to wait=u32 50) -> ()  [unwired: 1 out]
                    n207 = Or(x=w238, y=w239) -> (x .or. y?=w237:bool)
                  }
                }
                frame #7 {
                }
                frame #8 {
                }
              }
            }
          }
        }
        frame Enabled {
          n208 = global read "Robot Global Data.vi" "Autonomous Mode"() -> (w247:T7)
          n209 = case shown="\"No pot 1 bin\", Default" w247 {
            tunnel: w246 -> [_ _ _ _ w346 _ _]
            tunnel: w245 -> [_ _ _ _ w344 _ _]
            frame "1 Tote" {
              n210 = disable-structure shown="Disabled" {
                frame Disabled {
                  n211 = flat-sequence {
                    tunnel: w249 -> [w253]
                    tunnel: w248 -> [w252]
                    tunnel: w249 -> [w260]
                    tunnel: w248 -> [w259]
                    frame #0 {
                      n212 = call "calibrateArmEncoder.vi"() -> ()  [unwired: 12 in]
                    }
                    frame #1 {
                      n213 = call-poly <vilib>:"WPI_SolenoidSet.vi"("Value"=WPI_SolenoidValue."On", "SolenoidDevRef"=w252) -> ()  [unwired: 8 in, 2 out]
                      n214 = call-poly <vilib>:"WPI_SolenoidSet.vi"("Value"=WPI_SolenoidValue."Off", "SolenoidDevRef"=w253) -> ()  [unwired: 8 in, 2 out]
                    }
                    frame #2 {
                      n215 = call "RaiseElevator.vi"("Distance"=12.0) -> ()  [unwired: 11 in]
                    }
                    frame #3 {
                      n216 = call "runStraight1Tote.vi"("Distance In"=-70.0) -> ()  [unwired: 11 in]
                    }
                    frame #4 {
                      n217 = call "RaiseElevator.vi"("Distance"=-12.0) -> ()  [unwired: 11 in]
                    }
                    frame #5 {
                      n218 = call-poly <vilib>:"WPI_SolenoidSet.vi"("Value"=WPI_SolenoidValue."Off", "SolenoidDevRef"=w259) -> ()  [unwired: 8 in, 2 out]
                      n219 = call-poly <vilib>:"WPI_SolenoidSet.vi"("Value"=WPI_SolenoidValue."On", "SolenoidDevRef"=w260) -> ()  [unwired: 8 in, 2 out]
                    }
                  }
                  n220 = call <vilib>:"WPI_SolenoidRefNum Registry Get.vi"("refnum name"="solenoidOne") -> ("SolenoidDevRef"=w248:T8)  [unwired: 9 in, 1 out]
                  n221 = call <vilib>:"WPI_SolenoidRefNum Registry Get.vi"("refnum name"="solenoidTwo") -> ("SolenoidDevRef"=w249:T8)  [unwired: 9 in, 1 out]
                }
                frame Enabled {
                }
              }
            }
            frame "3 Tote" {
              n222 = disable-structure shown="Disabled" {
                frame Disabled {
                  n223 = flat-sequence {
                    tunnel: w264 -> [w268]
                    tunnel: w263 -> [w267]
                    tunnel: w263 -> [w279]
                    tunnel: w264 -> [w278]
                    tunnel: w263 -> [w284]
                    tunnel: w264 -> [w283]
                    tunnel: w263 -> [w295]
                    tunnel: w264 -> [w294]
                    tunnel: w263 -> [w300]
                    tunnel: w264 -> [w299]
                    tunnel: w263 -> [w307]
                    tunnel: w264 -> [w306]
                    frame #0 {
                      # "Drop arm"
                      n224 = call "calibrateArmEncoder.vi"() -> ()  [unwired: 12 in]
                    }
                    frame #1 {
                      # "Close Arm"
                      n225 = call-poly <vilib>:"WPI_SolenoidSet.vi"("Value"=WPI_SolenoidValue."Off", "SolenoidDevRef"=w267) -> ()  [unwired: 8 in, 2 out]
                      n226 = call-poly <vilib>:"WPI_SolenoidSet.vi"("Value"=WPI_SolenoidValue."On", "SolenoidDevRef"=w268) -> ()  [unwired: 8 in, 2 out]
                    }
                    frame #2 {
                      n227 = call "runStraight1Tote.vi"("Distance In"=63.65) -> ()  [unwired: 11 in]
                    }
                    frame #3 {
                      # "Raise Tote"
                      n228 = call "RaiseElevator.vi"("Distance"=19.0) -> ()  [unwired: 11 in]
                    }
                    frame #4 {
                      n229 = call "gyroTurn.vi"("Angle"=-90.0) -> ()  [unwired: 11 in]
                    }
                    frame #5 {
                      n230 = call "runStraight1Tote.vi"("Distance In"=51.0) -> ()  [unwired: 11 in]
                    }
                    frame #6 {
                      n231 = call "gyroTurn.vi"("Angle"=-90.0) -> ()  [unwired: 11 in]
                    }
                    frame #7 {
                      n232 = call "runStraight1Tote.vi"("Distance In"=28.65) -> ()  [unwired: 11 in]
                    }
                    frame #8 {
                      # "Lower tote onto \nsecond tote, open arm, \nlower arm, close arm,\nraise totes"
                      n233 = call "RaiseElevator.vi"("Distance"=-7.0) -> ()  [unwired: 11 in]
                    }
                    frame #9 {
                      n234 = call-poly <vilib>:"WPI_SolenoidSet.vi"("Value"=WPI_SolenoidValue."Off", "SolenoidDevRef"=w278) -> ()  [unwired: 8 in, 2 out]
                      n235 = call-poly <vilib>:"WPI_SolenoidSet.vi"("Value"=WPI_SolenoidValue."On", "SolenoidDevRef"=w279) -> ()  [unwired: 8 in, 2 out]
                    }
                    frame #10 {
                      n236 = call "RaiseElevator.vi"("Distance"=-7.0) -> ()  [unwired: 11 in]
                    }
                    frame #11 {
                      n237 = call-poly <vilib>:"WPI_SolenoidSet.vi"("Value"=WPI_SolenoidValue."On", "SolenoidDevRef"=w283) -> ()  [unwired: 8 in, 2 out]
                      n238 = call-poly <vilib>:"WPI_SolenoidSet.vi"("Value"=WPI_SolenoidValue."Off", "SolenoidDevRef"=w284) -> ()  [unwired: 8 in, 2 out]
                    }
                    frame #12 {
                      n239 = call "RaiseElevator.vi"("Distance"=19.0) -> ()  [unwired: 11 in]
                    }
                    frame #13 {
                      n240 = call "runStraight1Tote.vi"("Distance In"=-28.65) -> ()  [unwired: 11 in]
                    }
                    frame #14 {
                      n241 = call "gyroTurn.vi"("Angle"=90.0) -> ()  [unwired: 11 in]
                    }
                    frame #15 {
                      n242 = call "runStraight1Tote.vi"("Distance In"=51.0) -> ()  [unwired: 11 in]
                    }
                    frame #16 {
                      n243 = call "gyroTurn.vi"("Angle"=-90.0) -> ()  [unwired: 11 in]
                    }
                    frame #17 {
                      n244 = call "runStraight1Tote.vi"("Distance In"=28.65) -> ()  [unwired: 11 in]
                    }
                    frame #18 {
                      # "Lower tote onto \nthird tote, open arm,\nlower arm, close arm,\nraise totes"
                      n245 = call "RaiseElevator.vi"("Distance"=-7.0) -> ()  [unwired: 11 in]
                    }
                    frame #19 {
                      n246 = call-poly <vilib>:"WPI_SolenoidSet.vi"("Value"=WPI_SolenoidValue."Off", "SolenoidDevRef"=w294) -> ()  [unwired: 8 in, 2 out]
                      n247 = call-poly <vilib>:"WPI_SolenoidSet.vi"("Value"=WPI_SolenoidValue."On", "SolenoidDevRef"=w295) -> ()  [unwired: 8 in, 2 out]
                    }
                    frame #20 {
                      n248 = call "RaiseElevator.vi"("Distance"=-7.0) -> ()  [unwired: 11 in]
                    }
                    frame #21 {
                      n249 = call-poly <vilib>:"WPI_SolenoidSet.vi"("Value"=WPI_SolenoidValue."On", "SolenoidDevRef"=w299) -> ()  [unwired: 8 in, 2 out]
                      n250 = call-poly <vilib>:"WPI_SolenoidSet.vi"("Value"=WPI_SolenoidValue."Off", "SolenoidDevRef"=w300) -> ()  [unwired: 8 in, 2 out]
                    }
                    frame #22 {
                      n251 = call "RaiseElevator.vi"("Distance"=7.0) -> ()  [unwired: 11 in]
                    }
                    frame #23 {
                      n252 = call "runStraight1Tote.vi"("Distance In"=-107.0) -> ()  [unwired: 11 in]
                    }
                    frame #24 {
                      # "Lower totes,\nopen arm"
                      n253 = call "RaiseElevator.vi"("Distance"=-12.0) -> ()  [unwired: 11 in]
                    }
                    frame #25 {
                      n254 = call-poly <vilib>:"WPI_SolenoidSet.vi"("Value"=WPI_SolenoidValue."Off", "SolenoidDevRef"=w306) -> ()  [unwired: 8 in, 2 out]
                      n255 = call-poly <vilib>:"WPI_SolenoidSet.vi"("Value"=WPI_SolenoidValue."On", "SolenoidDevRef"=w307) -> ()  [unwired: 8 in, 2 out]
                    }
                    frame #26 {
                      n256 = call "runStraight1Tote.vi"("Distance In"=-6.0) -> ()  [unwired: 11 in]
                    }
                  }
                  n257 = call <vilib>:"WPI_SolenoidRefNum Registry Get.vi"("refnum name"="solenoidOne") -> ("SolenoidDevRef"=w263:T8)  [unwired: 9 in, 1 out]
                  n258 = call <vilib>:"WPI_SolenoidRefNum Registry Get.vi"("refnum name"="solenoidTwo") -> ("SolenoidDevRef"=w264:T8)  [unwired: 9 in, 1 out]
                }
                frame Enabled {
                }
              }
            }
            frame "2 Tote Middle" {
              n259 = disable-structure shown="Disabled" {
                frame Disabled {
                  n260 = call <vilib>:"WPI_SolenoidRefNum Registry Get.vi"("refnum name"="solenoidOne") -> ("SolenoidDevRef"=w312:T8)  [unwired: 9 in, 1 out]
                  n261 = call <vilib>:"WPI_SolenoidRefNum Registry Get.vi"("refnum name"="solenoidTwo") -> ("SolenoidDevRef"=w311:T8)  [unwired: 9 in, 1 out]
                  n262 = flat-sequence {
                    tunnel: w312 -> [w317]
                    tunnel: w311 -> [w316]
                    tunnel: w312 -> [w327]
                    tunnel: w311 -> [w326]
                    tunnel: w312 -> [w332]
                    tunnel: w311 -> [w331]
                    tunnel: w312 -> [w339]
                    tunnel: w311 -> [w338]
                    frame #0 {
                      # "Drop arm"
                      n263 = call "calibrateArmEncoder.vi"() -> ()  [unwired: 12 in]
                      n264 = call "runStraight1Tote.vi"("Distance In"=63.65) -> ()  [unwired: 11 in]
                    }
                    frame #1 {
                      # "Close Arm"
                      n265 = call-poly <vilib>:"WPI_SolenoidSet.vi"("Value"=WPI_SolenoidValue."On", "SolenoidDevRef"=w316) -> ()  [unwired: 8 in, 2 out]
                      n266 = call-poly <vilib>:"WPI_SolenoidSet.vi"("Value"=WPI_SolenoidValue."Off", "SolenoidDevRef"=w317) -> ()  [unwired: 8 in, 2 out]
                    }
                    frame #2 {
                    }
                    frame #3 {
                      # "Raise tote"
                      n267 = call "RaiseElevator.vi"("Distance"=19.0) -> ()  [unwired: 11 in]
                    }
                    frame #4 {
                      n268 = call "gyroTurn.vi"("Angle"=-90.0) -> ()  [unwired: 11 in]
                    }
                    frame #5 {
                      n269 = call "runStraight1Tote.vi"("Distance In"=51.0) -> ()  [unwired: 11 in]
                    }
                    frame #6 {
                      n270 = call "gyroTurn.vi"("Angle"=-90.0) -> ()  [unwired: 11 in]
                    }
                    frame #7 {
                      n271 = call "runStraight1Tote.vi"("Distance In"=28.65) -> ()  [unwired: 11 in]
                    }
                    frame #8 {
                      # "Lower tote onto \nsecond tote, open arm, \nlower arm, close arm,\nraise totes"
                      n272 = call "RaiseElevator.vi"("Distance"=-7.0) -> ()  [unwired: 11 in]
                    }
                    frame #9 {
                      n273 = call-poly <vilib>:"WPI_SolenoidSet.vi"("Value"=WPI_SolenoidValue."Off", "SolenoidDevRef"=w326) -> ()  [unwired: 8 in, 2 out]
                      n274 = call-poly <vilib>:"WPI_SolenoidSet.vi"("Value"=WPI_SolenoidValue."On", "SolenoidDevRef"=w327) -> ()  [unwired: 8 in, 2 out]
                    }
                    frame #10 {
                      n275 = call "RaiseElevator.vi"("Distance"=-7.0) -> ()  [unwired: 11 in]
                    }
                    frame #11 {
                      n276 = call-poly <vilib>:"WPI_SolenoidSet.vi"("Value"=WPI_SolenoidValue."On", "SolenoidDevRef"=w331) -> ()  [unwired: 8 in, 2 out]
                      n277 = call-poly <vilib>:"WPI_SolenoidSet.vi"("Value"=WPI_SolenoidValue."Off", "SolenoidDevRef"=w332) -> ()  [unwired: 8 in, 2 out]
                    }
                    frame #12 {
                      n278 = call "RaiseElevator.vi"("Distance"=7.0) -> ()  [unwired: 11 in]
                    }
                    frame #13 {
                      n279 = call "runStraight1Tote.vi"("Distance In"=-107.0) -> ()  [unwired: 11 in]
                    }
                    frame #14 {
                      # "Lower totes,\nopen arm"
                      n280 = call "RaiseElevator.vi"("Distance"=-12.0) -> ()  [unwired: 11 in]
                    }
                    frame #15 {
                      n281 = call-poly <vilib>:"WPI_SolenoidSet.vi"("Value"=WPI_SolenoidValue."Off", "SolenoidDevRef"=w338) -> ()  [unwired: 8 in, 2 out]
                      n282 = call-poly <vilib>:"WPI_SolenoidSet.vi"("Value"=WPI_SolenoidValue."On", "SolenoidDevRef"=w339) -> ()  [unwired: 8 in, 2 out]
                    }
                    frame #16 {
                      n283 = call "runStraight1Tote.vi"("Distance In"=-6.0) -> ()  [unwired: 11 in]
                    }
                  }
                }
                frame Enabled {
                }
              }
            }
            frame "3 Tote Spinny" {
            }
            frame "No pot 1 bin", Default {
              n284 = call <vilib>:"WPI_SolenoidRefNum Registry Get.vi"("refnum name"="solenoidOne") -> ("SolenoidDevRef"=w350:T8)  [unwired: 9 in, 1 out]
              n285 = call <vilib>:"WPI_SolenoidRefNum Registry Get.vi"("refnum name"="solenoidTwo") -> ("SolenoidDevRef"=w343:T8)  [unwired: 9 in, 1 out]
              n286 = call <vilib>:"WPI_MotorControlRefNum Registry Get.vi"("refnum name"="elevator") -> ("MotorControlDevRef"=w348:T10)  [unwired: 9 in, 1 out]
              n287 = flat-sequence {
                tunnel: w350 -> [w356]
                tunnel: w343 -> [w355]
                tunnel: [w354] -> w347
                tunnel: [w353] -> w345
                tunnel: w344 -> [w353]
                tunnel: w346 -> [w354]
                tunnel: w348 -> [w362]
                tunnel: w347 -> [w361]
                tunnel: w345 -> [w360]
                tunnel: w348 -> [w377]
                tunnel: _ -> [_]
                frame #0 {
                  n288 = call-poly <vilib>:"WPI_SolenoidSet.vi"("Value"=WPI_SolenoidValue."On", "SolenoidDevRef"=w356) -> ()  [unwired: 8 in, 2 out]
                  n289 = call-poly <vilib>:"WPI_SolenoidSet.vi"("Value"=WPI_SolenoidValue."Off", "SolenoidDevRef"=w355) -> ()  [unwired: 8 in, 2 out]
                  n290 = Wait (ms)(milliseconds to wait=u32 500) -> ()  [unwired: 1 out]
                }
                frame #1 {
                  n291 = while {
                    tunnel: w362 -> [w370]
                    tunnel: w361 -> [w368]
                    tunnel: w360 -> [w367]
                    i -> [w372]
                    stop <- w373 continue-if-true
                    n292 = call <vilib>:"WPI_MotorControlSetOutput.vi"("Output"=-0.5, "MotorControlDevRef"=w370) -> ()  [unwired: 7 in, 3 out]
                    n293 = call <vilib>:"WPI_SwitchRefNum Registry Get.vi"("refnum name"="topSwitch") -> ("error out"=w366:errorcluster, "SwitchDevRef"=w365:T3)  [unwired: 9 in]
                    n294 = Greater Or Equal?(x=w372, y=u32 5 ("milliseconds to wait")) -> (x >= y?=w374:bool)
                    n295 = call <vilib>:"WPI_SwitchGetLimitValue.vi"("error in (no error)"=w367, "SwitchDevRef"=w368) -> ()  [unwired: 7 in, 3 out]
                    n296 = call <vilib>:"WPI_SwitchGetLimitValue.vi"("error in (no error)"=w366, "SwitchDevRef"=w365) -> ("Switch Pressed"=w363:bool)  [unwired: 7 in, 2 out]
                    n297 = Wait (ms)(milliseconds to wait=u32 50) -> ()  [unwired: 1 out]
                    n298 = Or(x=w374, y=w363) -> (x .or. y?=w373:bool)
                  }
                }
                frame #2 {
                  n299 = call "runStraight1Tote.vi"("Distance In"=-95.0) -> ()  [unwired: 11 in]
                }
                frame #3 {
                  n300 = while {
                    tunnel: w377 -> [w378]
                    i -> [w380]
                    stop <- w382 stop-if-true
                    n301 = call <vilib>:"WPI_MotorControlSetOutput.vi"("Output"=0.5, "MotorControlDevRef"=w378) -> ()  [unwired: 7 in, 3 out]
                    n302 = call <vilib>:"WPI_SwitchRefNum Registry Get.vi"("refnum name"="bottomSwitch") -> ("error out"=w387:errorcluster, "SwitchDevRef"=w386:T3)  [unwired: 9 in]
                    n303 = call <vilib>:"WPI_SwitchGetLimitValue.vi"("error in (no error)"=w387, "SwitchDevRef"=w386) -> ("Switch Pressed"=w384:bool)  [unwired: 7 in, 2 out]
                    n304 = Greater Or Equal?(x=w380, y=5.0) -> (x >= y?=w383:bool)
                    n305 = Wait (ms)(milliseconds to wait=u32 50) -> ()  [unwired: 1 out]
                    n306 = Or(x=w383, y=w384) -> (x .or. y?=w382:bool)
                  }
                }
                frame #4 {
                }
                frame #5 {
                }
              }
            }
            frame "1 Bin" {
              n307 = disable-structure shown="Disabled" {
                frame Disabled {
                  n308 = call <vilib>:"WPI_SolenoidRefNum Registry Get.vi"("refnum name"="solenoidOne") -> ("SolenoidDevRef"=w390:T8)  [unwired: 9 in, 1 out]
                  n309 = call <vilib>:"WPI_SolenoidRefNum Registry Get.vi"("refnum name"="solenoidTwo") -> ("SolenoidDevRef"=w389:T8)  [unwired: 9 in, 1 out]
                  n310 = flat-sequence {
                    tunnel: w390 -> [w396]
                    tunnel: w389 -> [w394]
                    frame #0 {
                      n311 = Wait (ms)(milliseconds to wait=u32 500) -> ()  [unwired: 1 out]
                      n312 = call-poly <vilib>:"WPI_SolenoidSet.vi"("Value"=WPI_SolenoidValue."On", "SolenoidDevRef"=w396) -> ()  [unwired: 8 in, 2 out]
                      n313 = call-poly <vilib>:"WPI_SolenoidSet.vi"("Value"=WPI_SolenoidValue."Off", "SolenoidDevRef"=w394) -> ()  [unwired: 8 in, 2 out]
                    }
                    frame #1 {
                      n314 = call "RaiseElevator.vi"("Distance"=6.0) -> ()  [unwired: 11 in]
                    }
                    frame #2 {
                      n315 = call "runStraight1Tote.vi"("Distance In"=-70.0) -> ()  [unwired: 11 in]
                    }
                    frame #3 {
                      n316 = call "RaiseElevator.vi"("Distance"=-6.0) -> ()  [unwired: 11 in]
                    }
                  }
                }
                frame Enabled {
                }
              }
            }
            frame "Drive" {
              n317 = flat-sequence {
                frame #0 {
                  n318 = call "runStraight.vi"("Distance In"=36.0) -> ()  [unwired: 11 in]
                }
              }
            }
          }
        }
      }
    }
  }
